vi "Data.Init.vi"(8 "error in":errorcluster) -> (0 "error out":errorcluster, 3 "DVR":T1)   [LabVIEW 2020]
uses:
  _controls/data.ctl
  camera/camera.lvclass
  _controls/data.ref.ctl
  <vilib>/vision/Image Controls.llb/IMAQ Image.ctl
  _controls/state.ctl
  _controls/data.vars.ctl
  _controls/flip.ctl
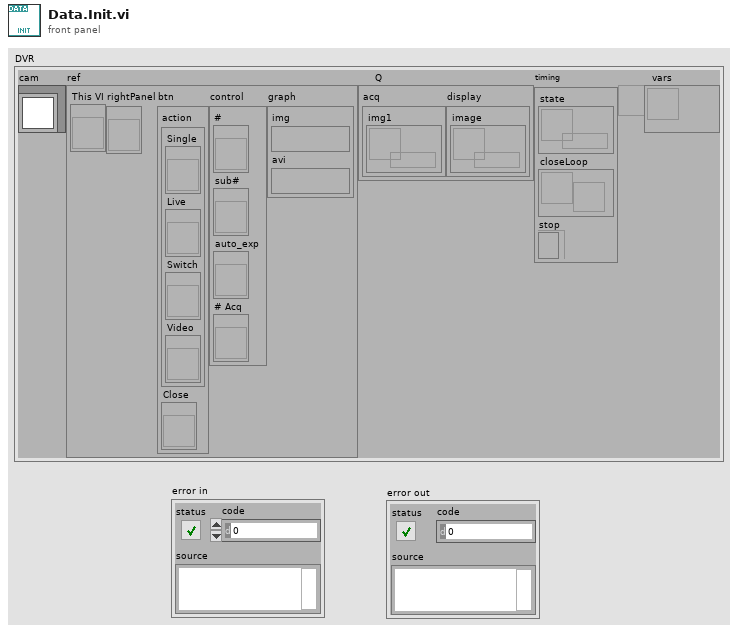
[diagram p1: front panel]
types:
  T1 = typedef "data.ctl" = cluster{"cam":refnum<class "camera.lvclass">, "ref":T2, "Q":cluster{"acq":cluster{"img1":refnum<queue>}, "display":cluster{"image":refnum<queue>}}, "timing":cluster{"state":refnum<queue>, "closeLoop":refnum<notifier>, "stop":refnum<k4>}, "vars":refnum<data-value>}
  T2 = typedef "data.ref.ctl" = cluster{"This VI":refnum<vi>, "rightPanel":refnum<vi>, "btn":cluster{"action":cluster{"Single":refnum<vi>, "Live":refnum<vi>, "Switch":refnum<vi>, "Video":refnum<vi>}, "Close":refnum<vi>}, "control":cluster{"#":refnum<vi>, "sub#":refnum<vi>, "auto_exp":refnum<vi>, "# Acq":refnum<vi>}, "graph":cluster{"img":T3, "avi":T3}}
  T3 = typedef "IMAQ Image.ctl" = refnum<image>
  T4 = typedef "data.vars.ctl" = cluster{"save":cluster{"base_folder":cluster{"Folder":path, "tif":bool, "jpg":bool}, "module":string, "#":u32, "sub#":u8, "save.op":enum16{"Full", "Light"}, "same?":bool, "Shift":enum16{"Single", "Leapfrog"}, "jpg?":bool, "flip":T5}, "acq":cluster{"# Acq":u16, "rotate":bool, "FPS":dbl}, "calib.manual":cluster{"BG":cluster{"Image":u16[][], "enabled?":bool}, "FF":cluster{"Image":u16[][], "enabled?":bool}}}
  T5 = typedef "flip.ctl" = cluster{"x":bool, "y":bool}
  T6 = typedef "state.ctl" = enum16{"-", "single", "video", "livePL", "PL"}
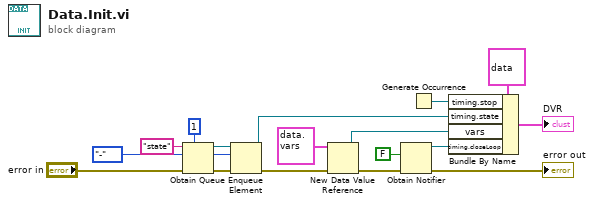
[diagram p0: block diagram]
diagram:
  w6 = state."-"
  n1 = Obtain Queue(max queue size (-1, unlimited)=1, name (unnamed)="state", element data type=w6, error in (no error)="error in") -> (queue out=w8:refnum<queue>, error out=w9:errorcluster)  [unwired: 1 in, 1 out]
  n2 = Enqueue Element(queue=w8, element=w6, error in (no error)=w9) -> (queue out=w7:refnum<queue>, error out=w4:errorcluster)  [unwired: 1 in, 1 out]
  "error out" <- w4
  n3 = New Data Value Reference(data value=T4 {"save"={"base_folder"={"Folder"=path "", "tif"=FALSE, "jpg"=FALSE}, "module"="", "#"=20, "sub#"=0, "save.op"=enum."Full", "same?"=FALSE, "Shift"=enum."Single", "jpg?"=FALSE, "flip"={"x"=FALSE, "y"=FALSE}}, "acq"={"# Acq"=100, "rotate"=FALSE, "FPS"=0.0}, "calib.manual"={"BG"={"Image"=[], "enabled?"=FALSE}, "FF"={"Image"=[], "enabled?"=FALSE}}}, error in=w4) -> (data value reference=w3:refnum<data-value>)  [unwired: 1 out]
  n4 = Obtain Notifier(notification data type=FALSE, error in (no error)=w4) -> (notifier out=w2:refnum<notifier>)  [unwired: 2 in, 2 out]
  n5 = Generate Occurrence() -> (w1:refnum<k4>)
  n6 = Bundle By Name(cluster=T1 {"cam"=refnum, "ref"={"This VI"=refnum, "rightPanel"=refnum, "btn"={"action"={"Single"=refnum, "Live"=refnum, "Switch"=refnum, "Video"=refnum}, "Close"=refnum}, "control"={"#"=refnum, "sub#"=refnum, "auto_exp"=refnum, "# Acq"=refnum}, "graph"={"img"=refnum, "avi"=refnum}}, "Q"={"acq"={"img1"=refnum}, "display"={"image"=refnum}}, "timing"={"state"=refnum, "closeLoop"=refnum, "stop"=refnum}, "vars"=refnum} ("DVR"), "timing.stop"=w1, "timing.state"=w7, "vars"=w3, "timing.closeLoop"=w2) -> (→"DVR":T1)
